vi "detectiongate2array.vi"(9 "T1_parameters":T1, 11 "correction_us":dbl) -> (0 "stop_read":u32[][](array[numeric]), 1 "start_read":u32[][](array[numeric]))   [LabVIEW 2014]
panel:
  out "stop-start":dbl[][](graph)
  # "* Every value of start_read and stop_read represents 2ns"
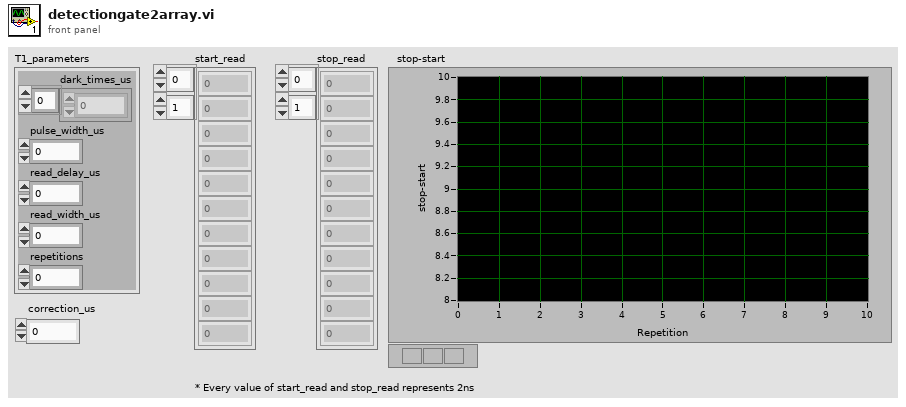
[diagram p1: front panel]
types:
  T1 = cluster{"dark_times_us":dbl[], "pulse_width_us":dbl, "read_delay_us":dbl, "read_width_us":dbl, "repetitions":i32}
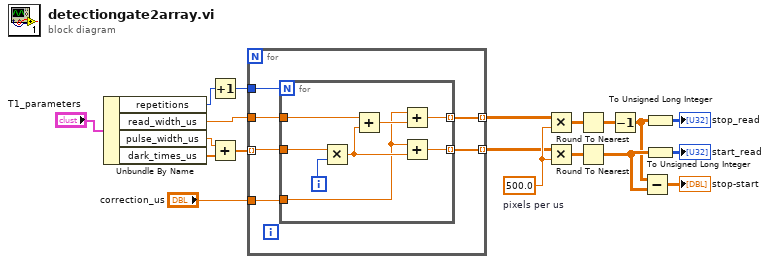
[diagram p0: block diagram]
diagram:
  w11 = 500.0  # pixels per us
  n1 = Unbundle By Name("T1_parameters") -> ("repetitions"=w12:i32, "read_width_us"=w17:dbl, "pulse_width_us"=w15:dbl, "dark_times_us"=w16:dbl[])
  n2 = Increment(x=w12) -> (x+1=w13:i32)
  n3 = Add(x=w15, y=w16) -> (x+y=w14:dbl[])
  n4 = for {
    tunnel: "correction_us" -> [w25]
    tunnel: w13 -> [w22]
    tunnel: w17 -> [w24]
    tunnel: w14 -> [w23] mode=indexing
    tunnel: [w21] -> w7 mode=indexing
    tunnel: [w20] -> w6 mode=indexing
    n5 = for {
      N: w22 -> [_]
      tunnel: w23 -> [w32]
      tunnel: w24 -> [w31]
      tunnel: [w27] -> w21 mode=indexing
      tunnel: [w26] -> w20 mode=indexing
      tunnel: w25 -> [w28]
      i -> [w33]
      n6 = Multiply(x=w32, y=w33) -> (x*y=w29:dbl)
      n7 = Add(x=w31, y=w29) -> (x+y=w30:dbl)
      n8 = Add(x=w28, y=w30) -> (x+y=w27:dbl)
      n9 = Add(x=w28, y=w29) -> (x+y=w26:dbl)
    }
  }
  n10 = Multiply(x=w7, y=w11) -> (x*y=w10:dbl[][])
  n11 = Multiply(x=w6, y=w11) -> (x*y=w9:dbl[][])
  n12 = Round To Nearest(number=w10) -> (nearest integer value=w5:dbl[][])
  n13 = Round To Nearest(number=w9) -> (nearest integer value=w4:dbl[][])
  n14 = Decrement(x=w5) -> (x-1=w3:dbl[][])
  n15 = Subtract(x=w3, y=w4) -> (x-y=→"stop-start":dbl[][])
  n16 = To Unsigned Long Integer(number=w3) -> (unsigned 32bit integer=→"stop_read":u32[][])
  n17 = To Unsigned Long Integer(number=w4) -> (unsigned 32bit integer=→"start_read":u32[][])
